vi "Core Actor - Send Actor Message.vi"(8 "error in (no error)":errorcluster, 9 "Value":string, 11 "Child_2_Class in":refnum<class "Console_Class.lvclass">) -> (0 "error out":errorcluster, 3 "Child_2_Class out":refnum<class "Console_Class.lvclass">)   [LabVIEW 2023, in "Console_Actor.lvlib" / "Console_Class.lvclass"]
uses:
  Console_Class.lvclass
  Child 2 - Ctrl - Trigger Event Cluster.ctl
  Usr Ev/Child_2 - Ctrl - Enum - Events (Temp).ctl
  Console_Class.lvclass/Console_Class.ctl
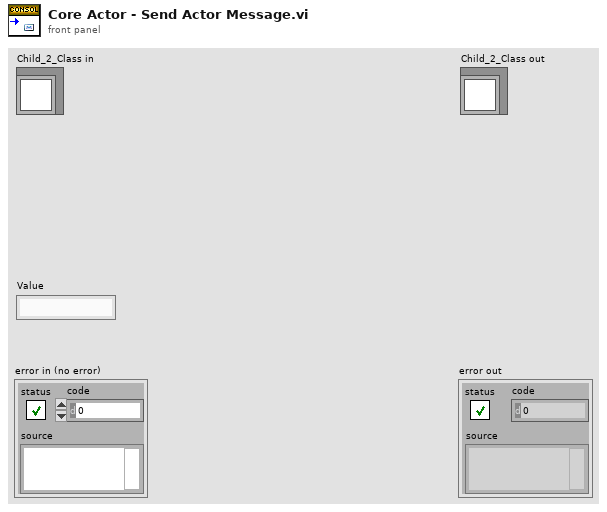
[diagram p1: front panel]
types:
  T1 = typedef "Console_Actor.lvlib/Console_Class.lvclass/Child 2 - Ctrl - Trigger Event Cluster.ctl" = cluster{"Events":T2, "Data":string}
  T2 = typedef "Console_Actor.lvlib/Console_Class.lvclass/Child_2 - Ctrl - Enum - Events (Temp).ctl" = enum16{"SEND MESSAGE Ev", "STOP_ACTOR Ev", "INIT_ACTOR Ev", "START Ev", "STOP Ev", "GET Ev", "SET Ev", "ERROR_HANDLER Ev", "RESET Ev", "T2 Ev", "T3 Ev", "T4 Ev"}
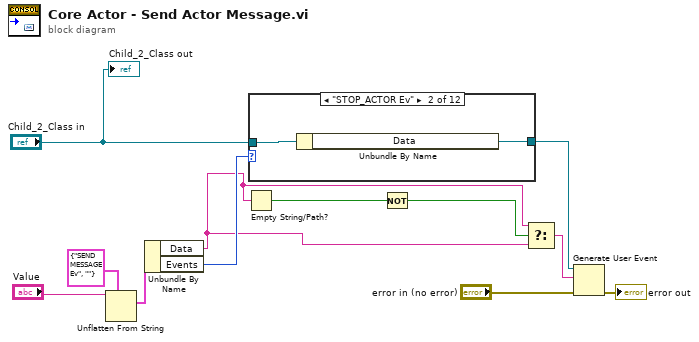
[diagram p0: block diagram]
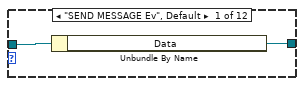
[diagram p2: hidden frame]
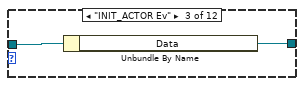
[diagram p3: hidden frame]
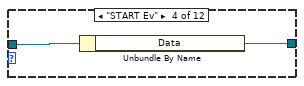
[diagram p4: hidden frame]
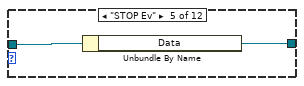
[diagram p5: hidden frame]
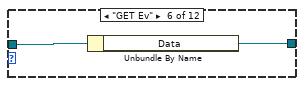
[diagram p6: hidden frame]
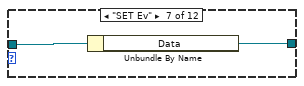
[diagram p7: hidden frame]
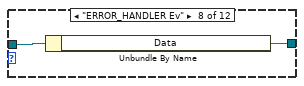
[diagram p8: hidden frame]
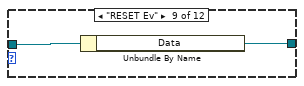
[diagram p9: hidden frame]
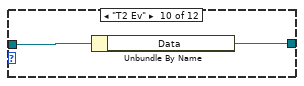
[diagram p10: hidden frame]
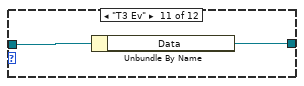
[diagram p11: hidden frame]
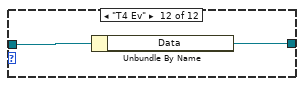
[diagram p12: hidden frame]
diagram:
  n1 = Unflatten From String(type=T1 {"Events"=enum."SEND MESSAGE Ev", "Data"=""} ("Child Trigger Event Cluster"), binary string="Value") -> (value=w3:T1)  [unwired: 3 in, 2 out]
  n2 = Unbundle By Name(w3) -> ("Data"=w1:string, "Events"=w2:T2)
  n3 = Empty String/Path?(string/path=w1) -> (empty?=w12:bool)
  n4 = case shown="\"STOP_ACTOR Ev\"" w2 {
    tunnel: "Child_2_Class in" -> [w14 w16 w18 w20 w22 w24 w26 w28 w30 w32 w34 w36]
    tunnel: [w13 w15 w17 w19 w21 w23 w25 w27 w29 w31 w33 w35] -> w10
    frame "SEND MESSAGE Ev", Default {
      n5 = Unbundle By Name(w14) -> ("Data"=w13:refnum<user-event>)
    }
    frame "STOP_ACTOR Ev" {
      n6 = Unbundle By Name(w16) -> ("Data"=w15:refnum<user-event>)
    }
    frame "INIT_ACTOR Ev" {
      n7 = Unbundle By Name(w18) -> ("Data"=w17:refnum<user-event>)
    }
    frame "START Ev" {
      n8 = Unbundle By Name(w20) -> ("Data"=w19:refnum<user-event>)
    }
    frame "STOP Ev" {
      n9 = Unbundle By Name(w22) -> ("Data"=w21:refnum<user-event>)
    }
    frame "GET Ev" {
      n10 = Unbundle By Name(w24) -> ("Data"=w23:refnum<user-event>)
    }
    frame "SET Ev" {
      n11 = Unbundle By Name(w26) -> ("Data"=w25:refnum<user-event>)
    }
    frame "ERROR_HANDLER Ev" {
      n12 = Unbundle By Name(w28) -> ("Data"=w27:refnum<user-event>)
    }
    frame "RESET Ev" {
      n13 = Unbundle By Name(w30) -> ("Data"=w29:refnum<user-event>)
    }
    frame "T2 Ev" {
      n14 = Unbundle By Name(w32) -> ("Data"=w31:refnum<user-event>)
    }
    frame "T3 Ev" {
      n15 = Unbundle By Name(w34) -> ("Data"=w33:refnum<user-event>)
    }
    frame "T4 Ev" {
      n16 = Unbundle By Name(w36) -> ("Data"=w35:refnum<user-event>)
    }
  }
  n17 = Not(x=w12) -> (.not. x?=w11:bool)
  n18 = Select(t=w1, s=w11, f=w1) -> (s? t:f=w9:string)
  n19 = Generate User Event(user event=w10, event data cluster=w9, error in="error in (no error)") -> (error out=→"error out":errorcluster)  [unwired: 1 in, 1 out]
  "Child_2_Class out" <- "Child_2_Class in"
